vi "XYZStage-Read position command.vi"(8 "error in (no error)":errorcluster, 10 "XY Stage config cluster":T1, 11 "UI ctrl refs":T2) -> (0 "error out":errorcluster, 2 "Coordinates":cluster{"X":sgl, "Y":sgl, "Z":sgl})   [LabVIEW 2013]
doc: "Reads the XYZ Stage coordinates"
uses:
  Typedefs/UI ctrl refs cluster.ctl
  Typedefs/Laser control knob.ctl
  Typedefs/Frame Size.ctl
  Typedefs/Plane Mode.ctl
  Typedefs/PMT control knob.ctl
  Typedefs/XY Stage config cluster.ctl
  <userlib>/_MGI/Application Control/MGI Change Detector/MGI Change Detector (T).vi
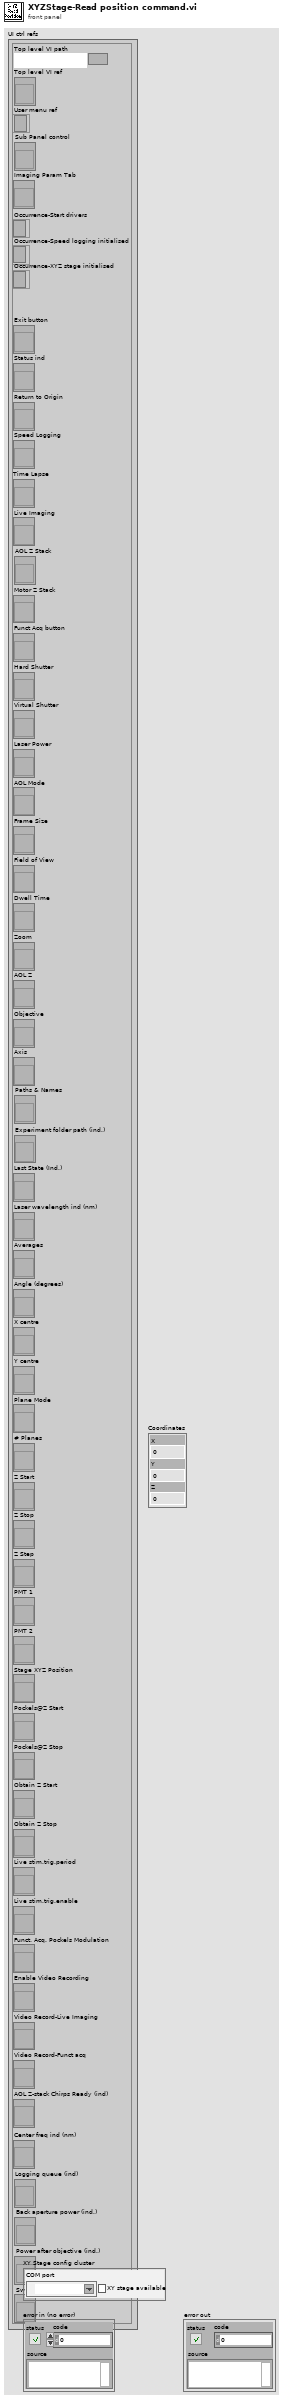
[diagram p1: front panel]
types:
  T1 = typedef "XY Stage config cluster.ctl" = cluster{"COM port":refnum<visa-resource-name>, "XY stage available":bool}
  T2 = typedef "UI ctrl refs cluster.ctl" = cluster{"Top level VI path":path, "Top level VI ref":refnum<vi>, "User menu ref":refnum<k9>, "Sub Panel control":refnum<vi>, "Imaging Param Tab":refnum<vi>, "Occurrence-Start drivers":refnum<k4>, "Occurrence-Speed logging initialised":refnum<k4>, "Occurrence-XYZ stage initialised":refnum<k4>, "Exit button":refnum<vi>, "Status ind":refnum<vi>, "Return to Origin":refnum<vi>, "Speed Logging":refnum<vi>, "Time Lapse":refnum<vi>, "Live Imaging":refnum<vi>, "AOL Z Stack":refnum<vi>, "Motor Z Stack":refnum<vi>, "Funct Acq button":refnum<vi>, "Hard Shutter":refnum<vi>, "Virtual Shutter":refnum<vi>, "Laser Power":refnum<vi>, "AOL Mode":refnum<vi>, "Frame Size":refnum<vi>, "Field of View":refnum<vi>, "Dwell Time":refnum<vi>, "Zoom":refnum<vi>, "AOL Z":refnum<vi>, "Objective":refnum<vi>, "Axis":refnum<vi>, "Paths & Names":refnum<vi>, "Experiment folder path (ind.)":refnum<vi>, "Last State (Ind.)":refnum<vi>, "Laser wavelength ind (nm)":refnum<vi>, "Averages":refnum<vi>, "Angle (degrees)":refnum<vi>, "X centre":refnum<vi>, "Y centre":refnum<vi>, "Plane Mode":refnum<vi>, "# Planes":refnum<vi>, "Z Start":refnum<vi>, "Z Stop":refnum<vi>, "Z Step":refnum<vi>, "PMT 1":refnum<vi>, "PMT 2":refnum<vi>, "Stage XYZ Position":refnum<vi>, "Pockels@Z Start":refnum<vi>, "Pockels@Z Stop":refnum<vi>, "Obtain Z Start":refnum<vi>, "Obtain Z Stop":refnum<vi>, "Live stim.trig.period":refnum<vi>, "Live stim.trig.enable":refnum<vi>, "Funct. Acq. Pockels Modulation":refnum<vi>, "Enable Video Recording":refnum<vi>, "Video Record-Live Imaging":refnum<vi>, "Video Record-Funct acq":refnum<vi>, "AOL Z-stack Chirps Ready (ind)":refnum<vi>, "Center freq ind (nm)":refnum<vi>, "Logging queue (ind)":refnum<vi>, "Back aperture power (ind.)":refnum<vi>, "Power after objective (ind.)":refnum<vi>, "Switch user":refnum<vi>}
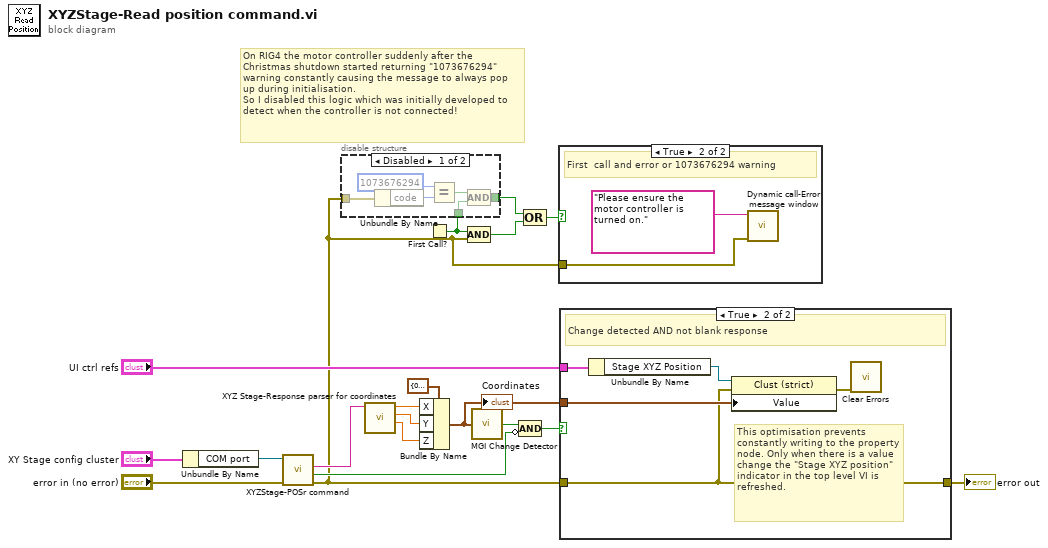
[diagram p0: block diagram]
diagram:
  # "On RIG4 the motor controller suddenly after the Christmas shutdown started returning \"1073676294\" warning constantly causing the message to always pop up during initialisation.\nSo I disabled this logic which was initially developed to detect when the controller is not connected!"
  n1 = Unbundle By Name("XY Stage config cluster") -> ("COM port"=w12:refnum<visa-resource-name>)
  n2 = call "XYZStage-POSr command.vi"("Error in"="error in (no error)", "VISA Refnum in"=w12) -> ("Error out"=w1:errorcluster, "Empty response string"=w7:bool, "read string"=w11:string)  [unwired: 6 in, 1 out]
  n3 = call "XYZ Stage-Response parser for coordinates.vi"("Filtered response string (no CR)"=w11) -> ("Z"=w18:sgl, "Y"=w17:sgl, "X"=w16:sgl)  [unwired: 8 in]
  n4 = Bundle By Name(cluster=cluster{"X":sgl, "Y":sgl, "Z":sgl} {"X"=0.0, "Y"=0.0, "Z"=0.0} ("Stage XYZ Position"), "X"=w16, "Y"=w17, "Z"=w18) -> (w9:cluster{"X":sgl, "Y":sgl, "Z":sgl})
  "Coordinates" <- w9
  n5 = First Call?() -> (First Call?: T/F=w4:bool)
  n6 = disable-structure shown="Disabled" {
    disable-tunnel: [w22 _] -> w5
    disable-tunnel: w4 -> [w21 _]
    disable-tunnel: w1 -> [w20 _]
    frame Disabled {
      n7 = Unbundle By Name(w20) -> ("code"=w25:i32)
      n8 = Equal?(x=1073676294, y=w25) -> (x = y?=w23:bool)
      n9 = Compound Arithmetic op=AND(w23, w21) -> (w22:bool)
    }
    frame Enabled {
    }
  }
  n10 = Compound Arithmetic op=AND(w4, w1) -> (w3:bool)
  n11 = call-poly <userlib>:"MGI Change Detector.vi"("Value"=w9) -> ("Changed?"=w8:bool)
  n12 = Compound Arithmetic op=AND(w8, invert w7) -> (w6:bool)
  n13 = Compound Arithmetic op=OR(w5, w3) -> (w2:bool)
  n14 = case shown="True" w2 {
    tunnel: w1 -> [_ w26]
    frame False {
    }
    frame True {
      # "First  call and error or 1073676294 warning"
      n15 = call "Dynamic call-Error message window.vi"("error in (no error)"=w26, "Error Message"="Please ensure the motor controller is turned on.") -> ()  [unwired: 9 in, 1 out]
    }
  }
  n16 = case shown="True" w6 {
    tunnel: [w28 w29] -> w19
    tunnel: w1 -> [w28 w29]
    tunnel: w9 -> [_ w33]
    tunnel: "UI ctrl refs" -> [_ w32]
    frame False {
      # "No change OR blank response"
    }
    frame True {
      # "This optimisation prevents constantly writing to the property node. Only when there is a value change the \"Stage XYZ position\" indicator in the top level VI is refreshed."
      # "Change detected AND not blank response"
      n17 = Unbundle By Name(w32) -> ("Stage XYZ Position"=w31:refnum<vi>)
      n18 = property on="Property Node" class="Clust (strict)"(reference=w31, error in=w29, "Value"=w33) -> (error out=w30:errorcluster)  [unwired: 1 out]
      n19 = call <vilib>:"Clear Errors.vi"("error in (no error)"=w30) -> ()  [unwired: 6 in, 1 out]
    }
  }
  "error out" <- w19
